vi "ztscopeM Horizontal.vi"(7 "Offset Time":dbl, 8 "error in":errorcluster, 9 "Sample Time":dbl=1.0, 10 "Sample Points":u32=1000, 11 "Instrument Handle In":i32) -> (0 "error out":errorcluster, 3 "Instrument Handle Out":i32)   [LabVIEW 2013]
doc: "Configure the horizontal and timebase settings."
uses:
  ztscopeM.dll
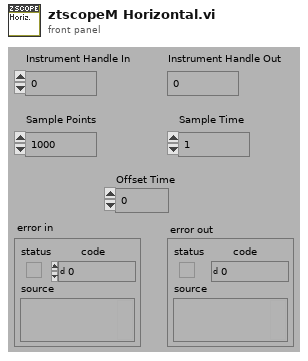
[diagram p1: front panel]
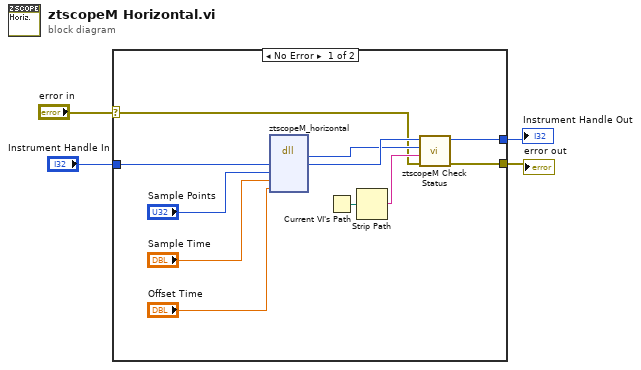
[diagram p0: block diagram]
diagram:
  n1 = case shown="No Error" "error in" {
    selector: "error in" -> [w8 w17]
    tunnel: [w7 w17] -> w1
    tunnel: "Instrument Handle In" -> [w15 w16]
    tunnel: [w6 w16] -> w3
    frame No Error {
      n2 = dll-call lib="C:/Program Files/National Instruments/instr.lib/ztscopem/ztscopeM.dll" fn="ztscopeM_horizontal"("instrumentHandle"=w15, "samplePoints"="Sample Points", "sampleTime"="Sample Time", "offsetTime"="Offset Time") -> (w9:i32, "instrumentHandle"=w10:i32)  [unwired: 6 in, 2 out]
      n3 = Current VI's Path() -> (path=w12:path)
      n4 = Strip Path(path=w12) -> (name=w11:string)  [unwired: 1 out]
      n5 = call "ztscopeM Check Status.vi"("error in"=w8, "name of VI"=w11, "status"=w9, "instrument handle in"=w10) -> ("error out"=w7:errorcluster, "instrument handle out"=w6:i32)  [unwired: 2 in]
    }
    frame Error {
    }
  }
  "Instrument Handle Out" <- w3
  "error out" <- w1
